vi "Available UART.vi"(8 "error in (no error)":errorcluster, 11 "VisaComms in":refnum<class "VisaComms.lvclass">) -> (0 "error out":errorcluster, 2 "Available UART":T1[](array[typedef]), 3 "VisaComms out":refnum<class "VisaComms.lvclass">)   [LabVIEW 2020, in "CTI.lvlib" / "VisaComms.lvclass"]
uses:
  VisaComms.lvclass
  Available UART.ctl
  UART Number.ctl
  GPIO Number.ctl
  VisaComms.lvclass/VisaComms.ctl
  Clean Visa Errors.vi
  CTI.lvlib
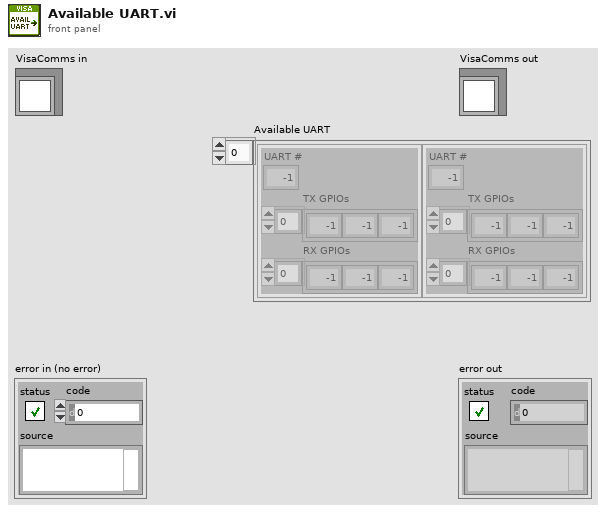
[diagram p1: front panel]
types:
  T1 = typedef "CTI.lvlib/Available UART.ctl" = cluster{"UART #":T2, "TX GPIOs":T3[], "RX GPIOs":T3[]}
  T2 = typedef "CTI.lvlib/UART Number.ctl" = i8
  T3 = typedef "CTI.lvlib/GPIO Number.ctl" = i8
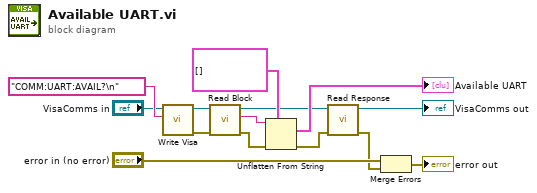
[diagram p0: block diagram]
diagram:
  n1 = call "Write Visa.vi"("write buffer"="COMM:UART:AVAIL?\n", "VisaComms in"="VisaComms in") -> ("error out"=w11:errorcluster, "VisaComms out"=w12:refnum<class "VisaComms.lvclass">)  [unwired: 7 in, 1 out]
  n2 = call "Read Block.vi"("error in (no error)"=w11, "VisaComms in"=w12) -> ("error out"=w14:errorcluster, "Block"=w10:string, "VisaComms out"=w2:refnum<class "VisaComms.lvclass">)  [unwired: 6 in, 1 out]
  n3 = Unflatten From String(type=T1[] [] ("Available UART"), binary string=w10, error in (no error)=w14) -> (value=→"Available UART":T1[], error out=w9:errorcluster)  [unwired: 2 in, 1 out]
  n4 = call "Read Response.vi"("error in (no error)"=w9, "VisaComms in"=w2) -> ("error out"=w3:errorcluster, "VisaComms out"=→"VisaComms out":refnum<class "VisaComms.lvclass">)  [unwired: 6 in, 2 out]
  n5 = Merge Errors("error in (no error)", w3) -> (→"error out":errorcluster)
